vi "RSZVB Diagram Area Title.vi"(7 "Title String":string, 8 "error in (no error)":errorcluster {"code" format="%.0x"}, 9 "Title (T: On)":bool=TRUE, 10 "Window (1)":i32=1, 11 "VISA session":refnum<visa-resource-name>) -> (0 "error out":errorcluster {"code" format="%.0x"}, 3 "dup VISA session":refnum<visa-resource-name>)   [LabVIEW 2011]
doc: "This VI defines a title for diagram area <Wnd>.\n\nTitle provides an input field for the title string. The title may comprise a practically unlimited number of characters and is centered in a line below the top of the diagram area.\n\nRemote-control command(s):\nDISPlay:WINDow<Wnd>:TITLe[:STATe] <Boolean>\nDISPlay:WINDow<Wnd>:TITLe:DATA '<string>'"
panel:
  # "On\nOff"
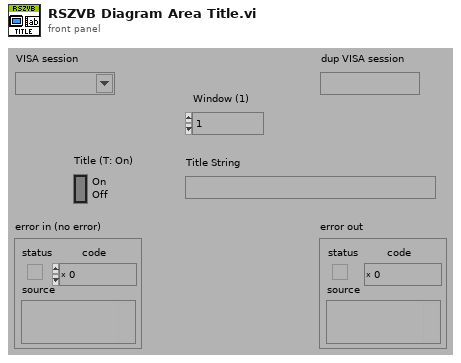
[diagram p1: front panel]
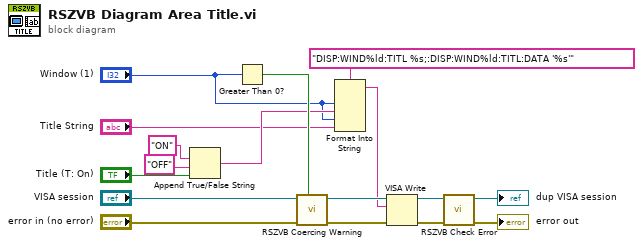
[diagram p0: block diagram]
diagram:
  n1 = Append True/False String(1:"Title (T: On)", 2:"OFF", 3:"ON") -> (0:w3:string)  [unwired: 1 in]
  n2 = Greater Than 0?(x="Window (1)") -> (x > 0?=w9:bool)
  n3 = call "RSZVB Coercing Warning.vi"("In Range?"=w9, "error in (no error)"="error in (no error)", "VISA session"="VISA session") -> ("error out"=w15:errorcluster, "dup VISA session"=w16:refnum<visa-resource-name>)  [unwired: 7 in]
  n4 = Format Into String(format string="DISP:WIND%ld:TITL %s;:DISP:WIND%ld:TITL:DATA '%s'", "Window (1)", w3, "Window (1)", "Title String") -> (resulting string=w12:string)  [unwired: 2 in, 1 out]
  n5 = VISA Write(VISA resource name=w16, write buffer=w12, error in (no error)=w15) -> (VISA resource name out=w13:refnum<visa-resource-name>, error out=w14:errorcluster)  [unwired: 1 out]
  n6 = call "RSZVB Check Error.vi"("error in (no error)"=w14, "VISA session"=w13) -> ("error out"=→"error out":errorcluster, "dup VISA session"=→"dup VISA session":refnum<visa-resource-name>)  [unwired: 8 in]
